vi "MRAWFileLoadSample.vi"() -> ()   [LabVIEW 8.6]
panel:
  in  "Stop":bool
  out "Picture":picture
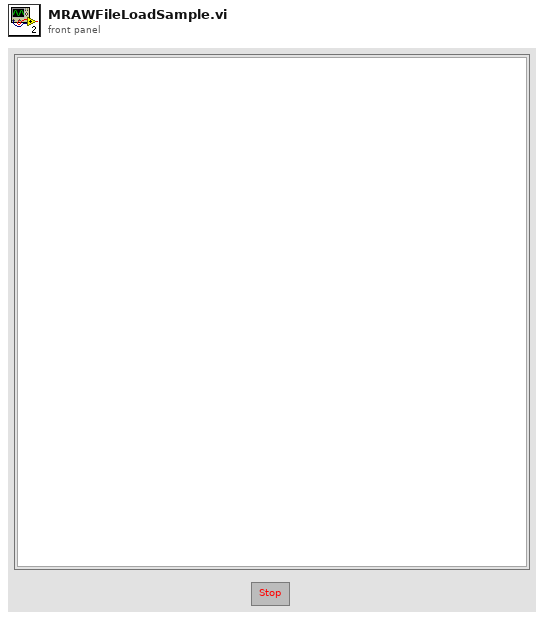
[diagram p1: front panel]
types:
  T1 = typedef "LVBoundsTypeDef.ctl" = cluster{"Width":u32, "Height":u32}
  T2 = cluster{"Width":i32, "Height":i32, "Byte Per Line":i32, "Real Bit Per Pixel":u16, "Interleave":i32}
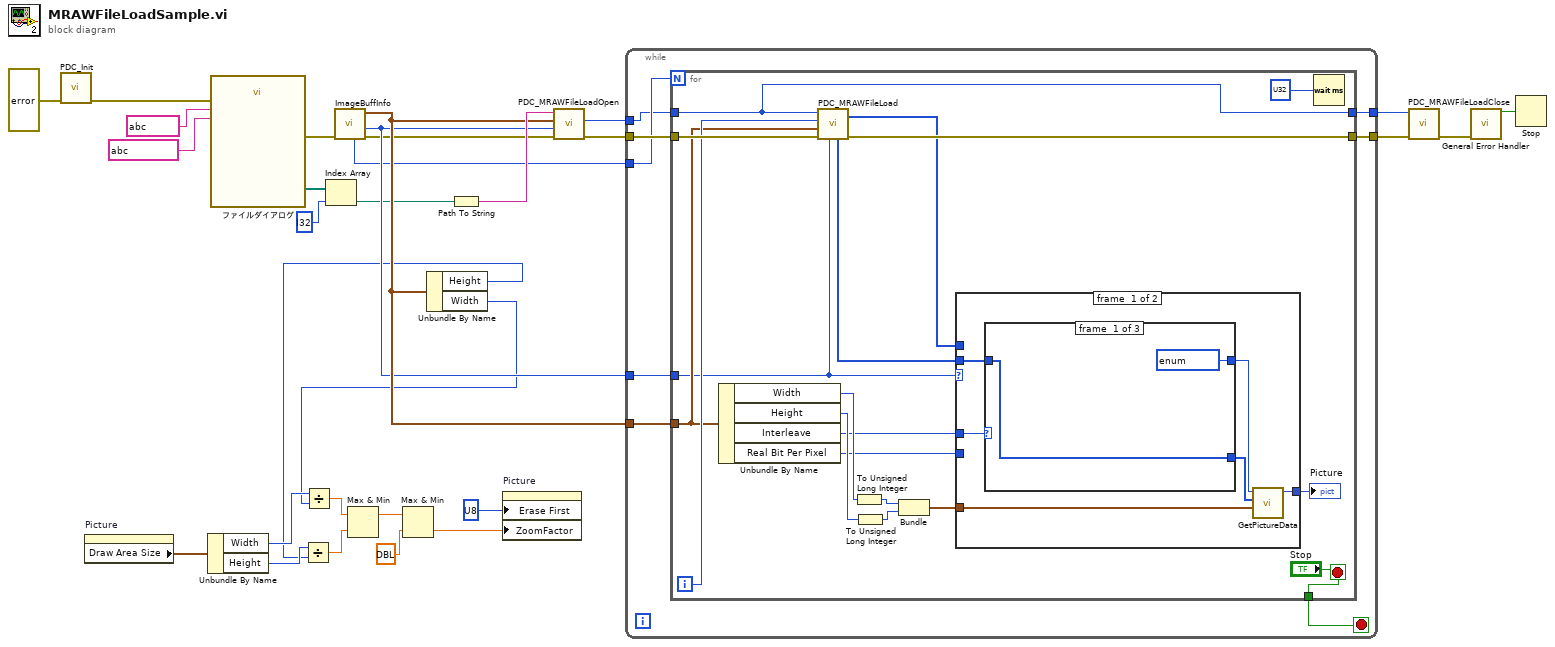
[diagram p0: block diagram]
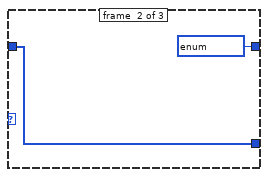
[diagram p2: hidden frame]
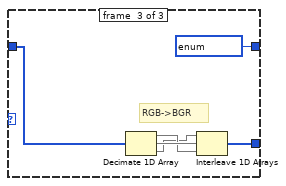
[diagram p3: hidden frame]
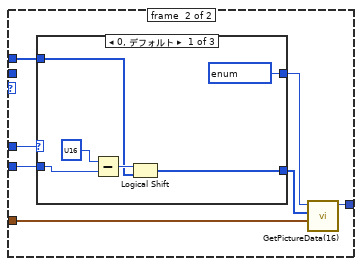
[diagram p4: hidden frame]
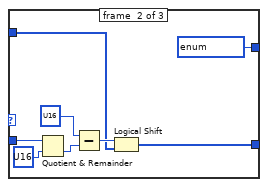
[diagram p5: hidden frame]
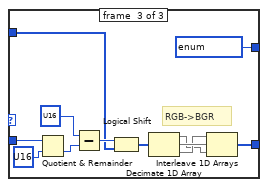
[diagram p6: hidden frame]
diagram:
  n1 = call "PDC_Init.vi"("error in (no error)"=errorcluster ?) -> ("error out"=w27:errorcluster)  [unwired: 8 in, 2 out]
  n2 = property on="Picture" class="Pict"() -> ("Draw Area Size"=w4:T1)  [unwired: 2 in, 2 out]
  n3 = Unbundle By Name(w4) -> ("Width"=w13:u32, "Height"=w12:u32)
  n4 = call "ファイルダイアログ"("error in"=w27, "pattern (all files)"=string ?, "pattern label"=string ?) -> ("selected paths"=w25:path[], "error out"=w26:errorcluster)  [unwired: 9 in, 2 out]
  n5 = Index Array(array=w25, index=i32 ? ("指標")) -> (element=w3:path)
  n6 = call "ImageBuffInfo.vi"("error in (no error)"=w26) -> ("error out"=w2:errorcluster, "MRaw Bit Depth"=w15:u32, "Image Buff Info"=w21:T2, "Total Frame"=w1:u32)  [unwired: 6 in, 1 out]
  n7 = Unbundle By Name(w21) -> ("Height"=w5:i32, "Width"=w6:i32)
  n8 = Divide(x=w12, y=w5) -> (x/y=w10:dbl)
  n9 = Divide(x=w13, y=w6) -> (x/y=w11:dbl)
  n10 = Max & Min(x=w11, y=w10) -> (max(x,y)=w9:dbl)  [unwired: 1 out]
  n11 = Max & Min(x=w9, y=dbl ?) -> (min(x,y)=w7:dbl)  [unwired: 1 out]
  n12 = Path To String(path=w3) -> (string=w23:string)
  n13 = property on="Picture" class="Pict"("Erase First"=u8 ? ("最初に削除"), "ZoomFactor"=w7) -> ()  [unwired: 2 in, 2 out]
  n14 = call "PDC_MRAWFileLoadOpen.vi"("FileName"=w23, "ImageBuffInfo"=w21, "MRawBitDepth"=w15, "error in (no error)"=w2) -> ("FileNo"=w22:u32, "error out"=w16:errorcluster)  [unwired: 1 in, 2 out]
  n15 = while {
    tunnel: w22 -> [w31]
    tunnel: w21 -> [w38]
    tunnel: w15 -> [w37]
    tunnel: w16 -> [w36]
    tunnel: [w35] -> w19
    tunnel: w1 -> [w33]
    tunnel: [w32] -> w17
    stop <- w34 stop-if-true
    n16 = for {
      N: w33 -> [_]
      tunnel: w31 -> [w41]
      tunnel: w38 -> [w40]
      tunnel: w37 -> [w39]
      tunnel: w36 -> [w45]
      tunnel: [w46] -> w35
      tunnel: ["Stop"] -> w34
      tunnel: [w41] -> w32
      i -> [w42]
      stop <- "Stop" stop-if-true
      n17 = Unbundle By Name(w40) -> ("Width"=w53:i32, "Height"=w52:i32, "Interleave"=w48:i32, "Real Bit Per Pixel"=w47:u16)
      n18 = call "PDC_MRAWFileLoad.vi"("MRawBitDepth"=w39, "error in (no error)"=w45, "ImageBuffInfo"=w40, "FrameNo"=w42, "FileNo"=w41) -> ("error out"=w46:errorcluster, "Data(8Bit)"=w43:u8[], "Data(16Bit)"=w44:u16[])  [unwired: 2 in, 2 out]
      n19 = To Unsigned Long Integer(number=w53) -> (unsigned 32bit integer=w49:u32)
      n20 = To Unsigned Long Integer(number=w52) -> (unsigned 32bit integer=w51:u32)
      n21 = Bundle(w49, w51) -> (w54:cluster{u32, u32})  [unwired: 1 in]
      n22 = case shown="1..3, デフォルト" w39 {
        tunnel: w43 -> [w57 _]
        tunnel: [w61 w79] -> w55
        tunnel: w44 -> [_ w74]
        tunnel: w54 -> [w62 w78]
        tunnel: w48 -> [w58 w77]
        tunnel: w47 -> [_ w75]
        frame #0 {
          n23 = case shown="2" w58 {
            tunnel: [enum16{"MONO", "COLOR"} ? ("ColorType") enum16{"MONO", "COLOR"} ? ("ColorType") enum16{"MONO", "COLOR"} ? ("ColorType")] -> w59
            tunnel: [w63 w65 w71] -> w60
            tunnel: w57 -> [w63 w65 w70]
            frame #0 {
            }
            frame #1 {
            }
            frame #2 {
              # "RGB->BGR"
              n24 = Decimate 1D Array(w70) -> (w68:u8[], w69:u8[], w67:u8[])
              n25 = Interleave 1D Arrays(w67, w69, w68) -> (w71:u8[])
            }
          }
          n26 = call "GetPictureData.vi"("Resolution"=w62, "Data(8Bit)"=w60, "ColorType"=w59) -> ("new picture"=w61:picture)  [unwired: 4 in]
        }
        frame #1 {
          n27 = case shown="0, デフォルト" w77 {
            tunnel: [enum16{"MONO", "COLOR"} ? ("ColorType") enum16{"MONO", "COLOR"} ? ("ColorType") enum16{"MONO", "COLOR"} ? ("ColorType")] -> w76
            tunnel: w75 -> [w82 w88 w101]
            tunnel: w74 -> [w83 w90 w99]
            tunnel: [w80 w86 w97] -> w73
            frame #0 {
              n28 = Subtract(x=u16 ?, y=w82) -> (x-y=w84:u16)
              n29 = Logical Shift(y=w84, x=w83) -> (x << y=w80:u16[])
            }
            frame #1 {
              n30 = Quotient & Remainder(x=w88, y=u16 ?) -> (floor(x/y)=w89:u16)  [unwired: 1 out]
              n31 = Subtract(x=u16 ?, y=w89) -> (x-y=w91:u16)
              n32 = Logical Shift(y=w91, x=w90) -> (x << y=w86:u16[])
            }
            frame #2 {
              # "RGB->BGR"
              n33 = Quotient & Remainder(x=w101, y=u16 ?) -> (floor(x/y)=w102:u16)  [unwired: 1 out]
              n34 = Subtract(x=u16 ?, y=w102) -> (x-y=w103:u16)
              n35 = Logical Shift(y=w103, x=w99) -> (x << y=w98:u16[])
              n36 = Decimate 1D Array(w98) -> (w94:u16[], w96:u16[], w95:u16[])
              n37 = Interleave 1D Arrays(w95, w96, w94) -> (w97:u16[])
            }
          }
          n38 = call "GetPictureData(16).vi"("Resolution"=w78, "Data(16Bit)"=w73, "ColorType"=w76) -> ("new picture"=w79:picture)  [unwired: 4 in]
        }
      }
      "Picture" <- w55
      n39 = Wait (ms)(milliseconds to wait=u32 ? ("ミリ秒待機時間")) -> ()  [unwired: 1 out]
    }
  }
  n40 = call "PDC_MRAWFileLoadClose.vi"("error in (no error)"=w19, "FileNo"=w17) -> ("error out"=w18:errorcluster)  [unwired: 7 in, 2 out]
  n41 = call <vilib>:"General Error Handler.vi"("error in (no error)"=w18) -> ("error?"=w20:bool)  [unwired: 10 in, 4 out]
  n42 = Stop(stop? (T)=w20) -> ()
